vi "cross correlation trial.vi"() -> ()   [LabVIEW 2012, in "Thorcam.lvclass"]
uses:
  Thorcam.lvclass
  <vilib>/Analysis/baseanly.llb/Mean (DBL).vi
  <vilib>/vision/NI_Vision_Development_Module.lvlib
  <vilib>/Analysis/NI_AALBase.lvlib
panel:
  out "System XY Graph":cluster{i32[], i32[]}(graph)
  out "mean calculation time (ms)":dbl format="%0.2f"
  out "(x,y) of max":i32[](array[numeric])
  out "y axis average":sgl[](graph)
  out "x axis average":sgl[](graph)
  out "Rob":T1(plugin-control)
  out "Roy":T1(plugin-control)
  out "pixel position of max of CC":i32[](graph)
  out "error out":errorcluster
  out "CC":T1(plugin-control)
  in  "path 2":path
  in  "path":path
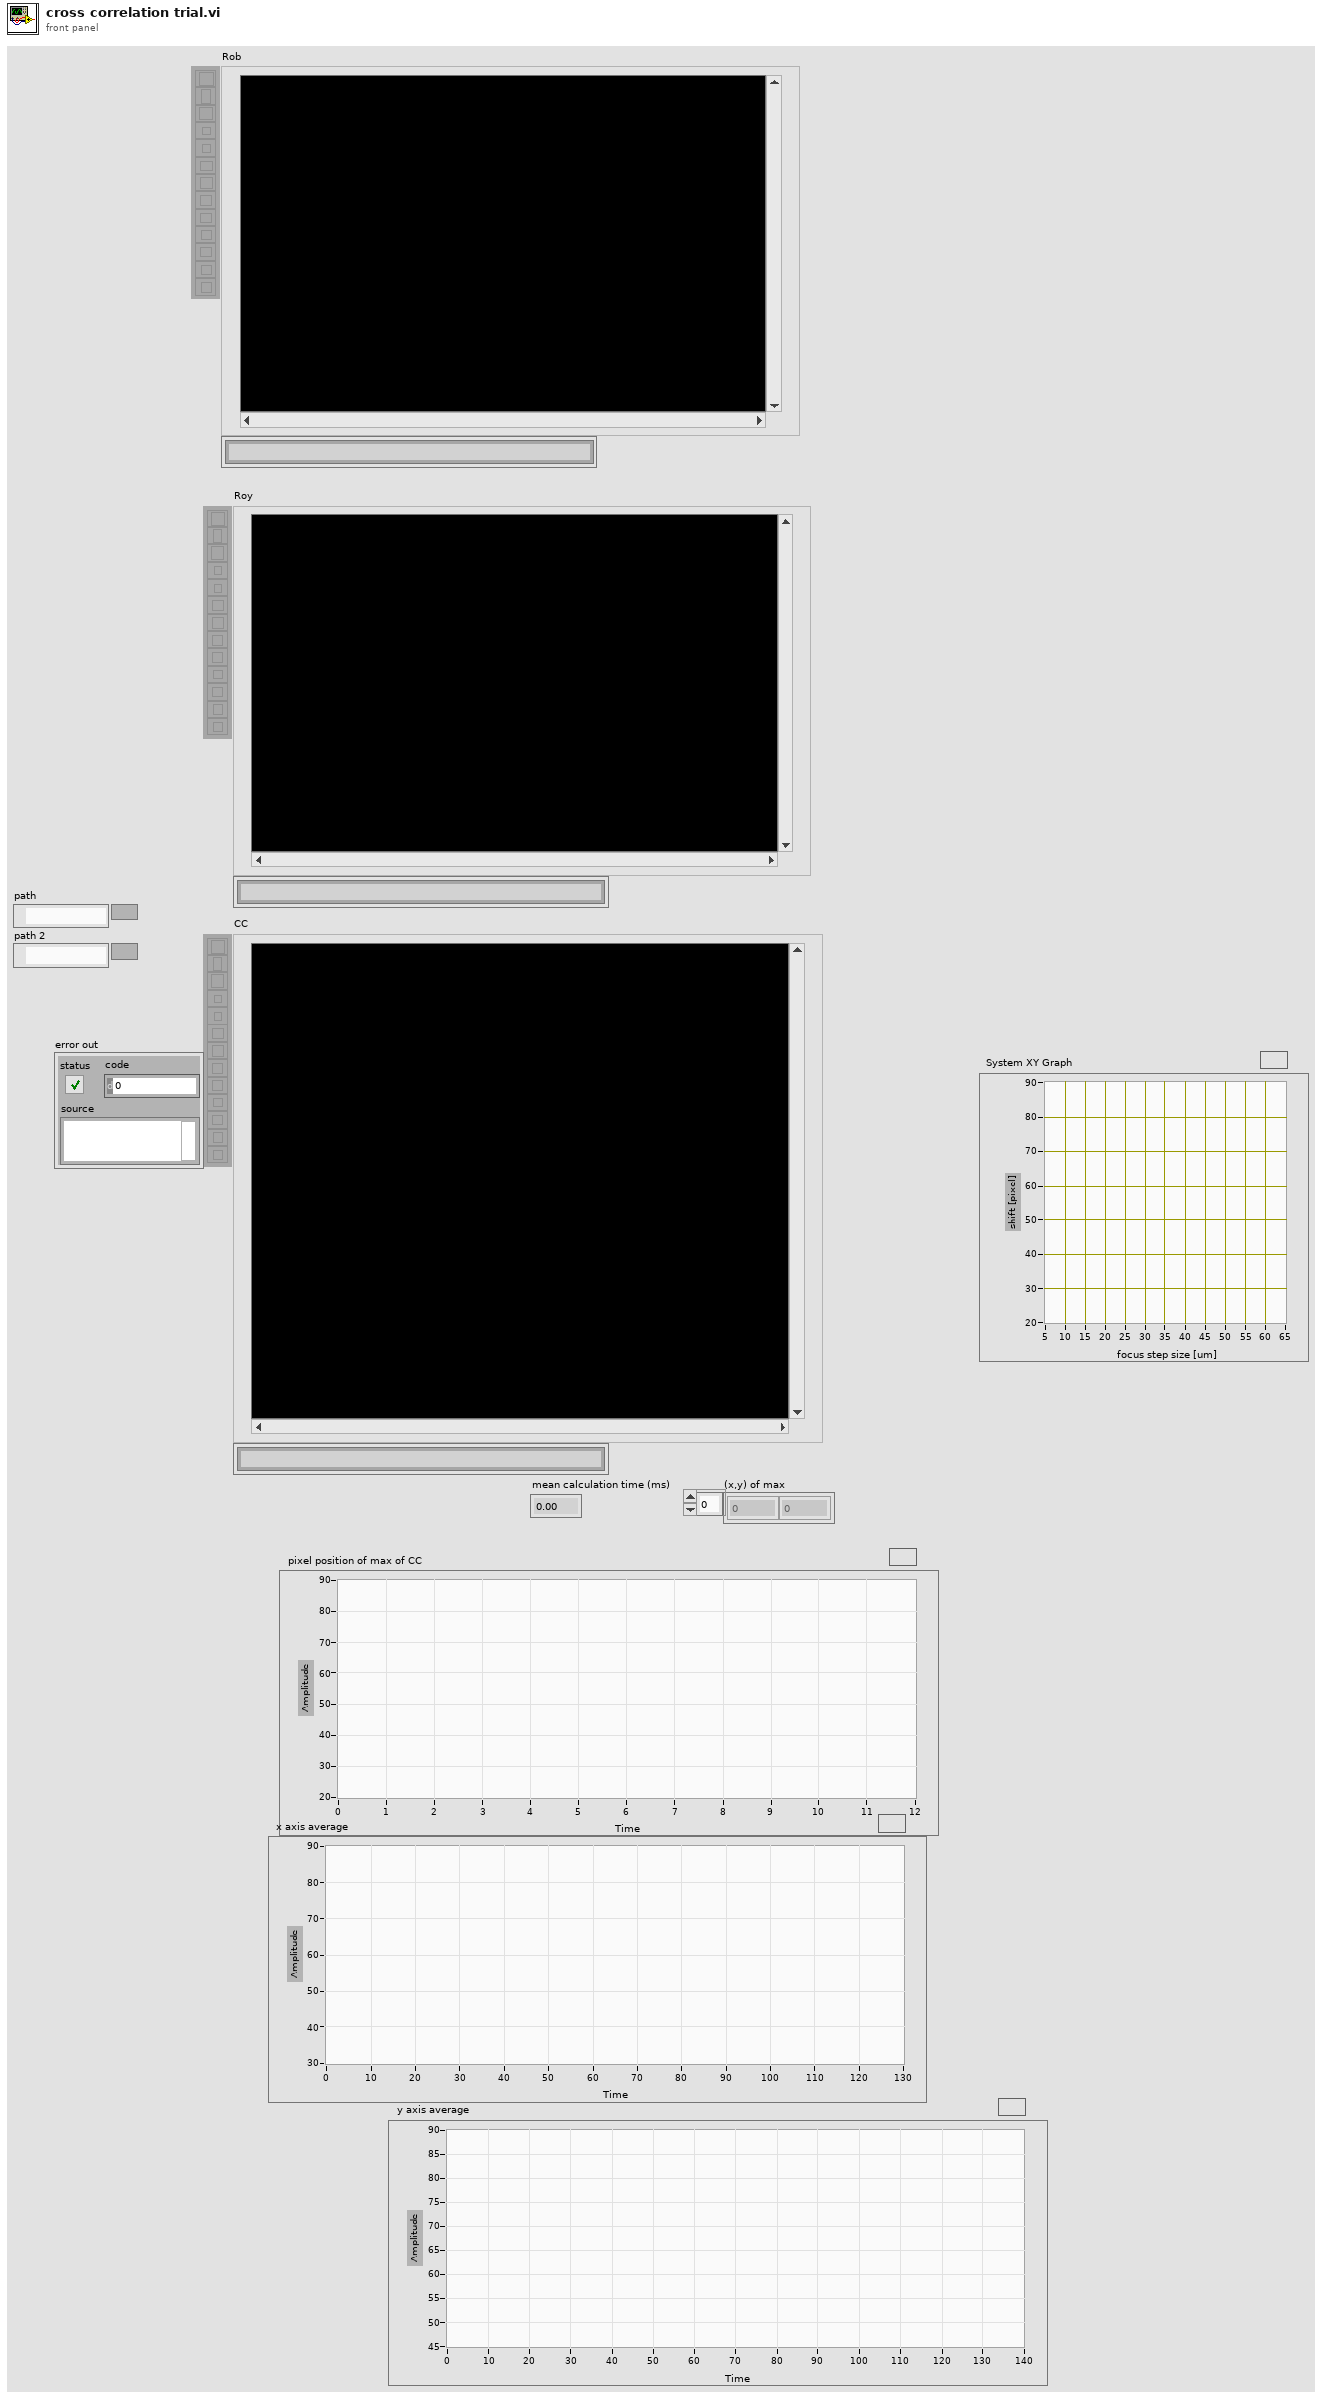
[diagram p1: front panel]
types:
  T1 = typedef "IMAQ Image.ctl" = refnum<image>
  T2 = cluster{"X Size":i32, "Y Size":i32, "Order #":i32}
  T3 = cluster{"histogram":u32[], "Minimal Value":sgl, "Maximal Value":sgl, "Starting Value":sgl, "Interval Width":sgl, "Mean Value":sgl, "Standard  Variation":sgl, "Area (pixels)":i32}
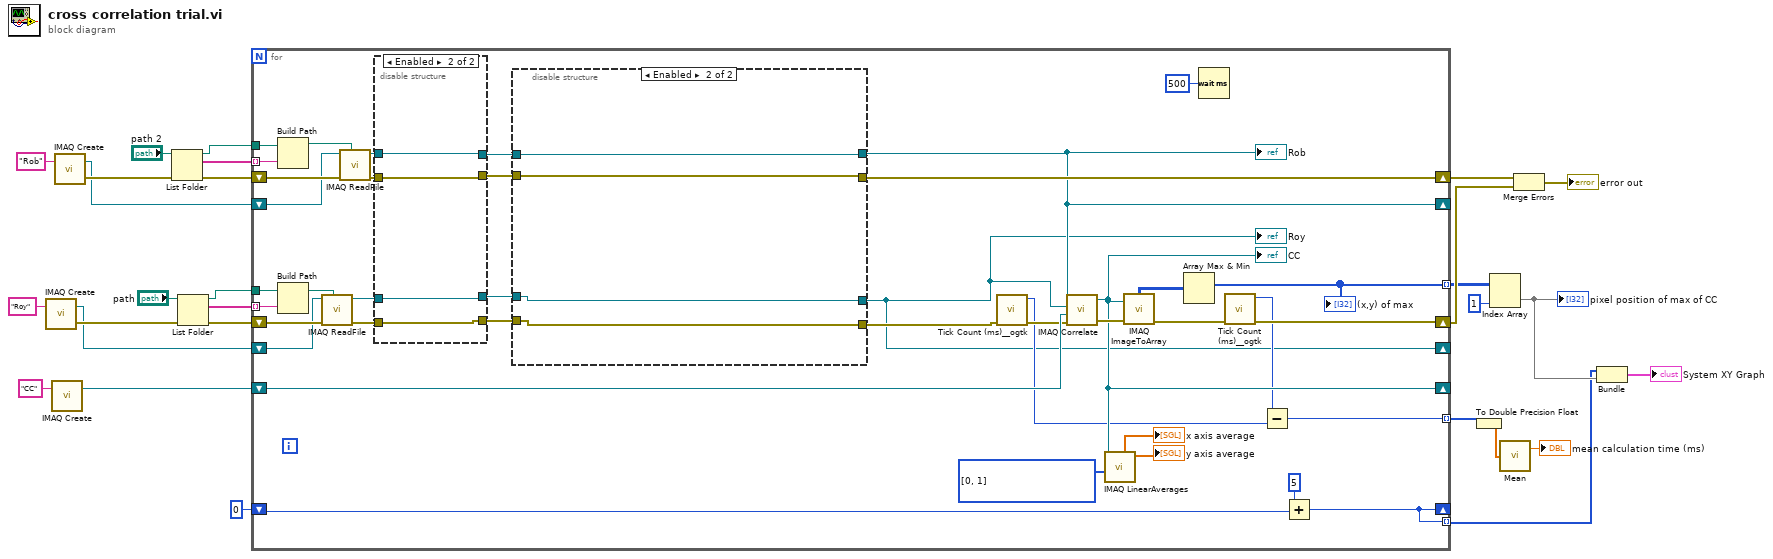
[diagram p0: block diagram]
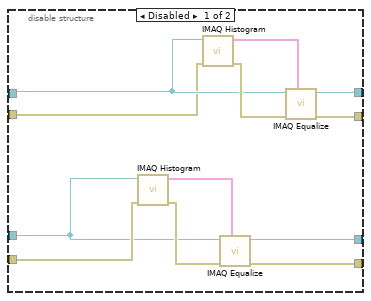
[diagram p2: hidden frame]
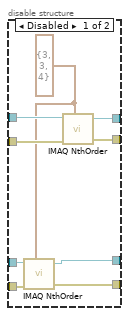
[diagram p3: hidden frame]
diagram:
  n1 = call "IMAQ Create"("Image Name"="Roy") -> ("New Image"=w18:T1, "error out"=w20:errorcluster)  [unwired: 4 in]
  n2 = call "IMAQ Create"("Image Name"="CC") -> ("New Image"=w10:T1)  [unwired: 4 in, 1 out]
  n3 = call "IMAQ Create"("Image Name"="Rob") -> ("New Image"=w21:T1, "error out"=w24:errorcluster)  [unwired: 4 in]
  n4 = List Folder(path="path 2", error in=w24) -> (path out=w22:path, filenames=w25:string[], error out=w23:errorcluster)  [unwired: 2 in, 1 out]
  n5 = List Folder(path="path", error in=w20) -> (path out=w17:path, filenames=w26:string[], error out=w19:errorcluster)  [unwired: 2 in, 1 out]
  n6 = for {
    tunnel: w26 -> [w61] mode=indexing
    tunnel: w25 -> [w67] mode=indexing
    tunnel: w22 -> [w66]
    shift-right: [w36] -> w14
    shift-left: w23 -> [w68]
    shift-right: [w35] -> _
    shift-left: w21 -> [w64]
    tunnel: w17 -> [w60]
    shift-right: [w47] -> w13
    shift-left: w19 -> [w63]
    shift-right: [w32] -> _
    shift-left: w18 -> [w62]
    tunnel: [w54] -> w9 mode=indexing
    shift-right: [w52] -> _
    shift-left: w10 -> [w55]
    tunnel: [w44] -> w7 mode=indexing
    shift-right: [w41] -> _
    shift-left: 0 -> [w42]
    tunnel: [w41] -> w2 mode=indexing
    w53 = i32[] [0, 1] items=["X Axis Averages", "Y Axis Averages", "X + Y Axis Averages", "X - Y Axis Averages"] ("Averages")
    n7 = Build Path(base path=w66, name or relative path=w67) -> (appended path=w65:path)
    n8 = Build Path(base path=w60, name or relative path=w61) -> (appended path=w59:path)
    n9 = call "IMAQ ReadFile"("File Path"=w59, "error in (no error)"=w63, "Image"=w62) -> ("error out"=w38:errorcluster, "Image Out"=w37:T1)  [unwired: 4 in, 3 out]
    n10 = call "IMAQ ReadFile"("File Path"=w65, "error in (no error)"=w68, "Image"=w64) -> ("error out"=w40:errorcluster, "Image Out"=w39:T1)  [unwired: 4 in, 3 out]
    n11 = disable-structure shown="Enabled" {
      disable-tunnel: w40 -> [w93 w96]
      disable-tunnel: w39 -> [w92 w97]
      disable-tunnel: w38 -> [w91 w94]
      disable-tunnel: w37 -> [w90 w95]
      disable-tunnel: [w88 w94] -> w34
      disable-tunnel: [w87 w95] -> w31
      disable-tunnel: [w86 w97] -> w30
      disable-tunnel: [w85 w96] -> w29
      frame Disabled {
        w89 = T2 {"X Size"=3, "Y Size"=3, "Order #"=4} ("Size & Order #")
        n12 = call "IMAQ NthOrder"("Image Src"=w90, "Size & Order #"=w89, "error in (no error)"=w91) -> ("Image Dst Out"=w87:T1, "error out"=w88:errorcluster)  [unwired: 4 in]
        n13 = call "IMAQ NthOrder"("Image Src"=w92, "Size & Order #"=w89, "error in (no error)"=w93) -> ("Image Dst Out"=w86:T1, "error out"=w85:errorcluster)  [unwired: 4 in]
      }
      frame Enabled {
      }
    }
    n14 = disable-structure shown="Enabled" {
      disable-tunnel: [w80 w83] -> w36
      disable-tunnel: [w79 w84] -> w35
      disable-tunnel: w34 -> [w76 w81]
      disable-tunnel: [w74 w81] -> w33
      disable-tunnel: [w72 w82] -> w32
      disable-tunnel: w31 -> [w71 w82]
      disable-tunnel: w30 -> [w70 w84]
      disable-tunnel: w29 -> [w69 w83]
      frame Disabled {
        n15 = call "IMAQ Histogram"("error in (no error)"=w76, "Image"=w71) -> ("error out"=w75:errorcluster, "Histogram Report"=w73:T3)  [unwired: 8 in]
        n16 = call "IMAQ Histogram"("error in (no error)"=w69, "Image"=w70) -> ("error out"=w78:errorcluster, "Histogram Report"=w77:T3)  [unwired: 8 in]
        n17 = call "IMAQ Equalize"("Histogram Report"=w73, "error in (no error)"=w75, "Image Src"=w71) -> ("error out"=w74:errorcluster, "Image Dst Out"=w72:T1)  [unwired: 7 in]
        n18 = call "IMAQ Equalize"("Histogram Report"=w77, "error in (no error)"=w78, "Image Src"=w70) -> ("error out"=w80:errorcluster, "Image Dst Out"=w79:T1)  [unwired: 7 in]
      }
      frame Enabled {
      }
    }
    "Roy" <- w32
    "Rob" <- w35
    n19 = call <userlib>:"Tick Count (ms)__ogtk.vi"("error in (no error)"=w33) -> ("error out"=w49:errorcluster, "millisecond timer value"=w45:u32)  [unwired: 9 in]
    n20 = call "IMAQ Correlate"("Image Src"=w35, "Image Template"=w32, "Image Dst"=w55, "error in (no error)"=w49) -> ("Image Dst Out"=w52:T1, "error out"=w58:errorcluster)  [unwired: 3 in]
    "CC" <- w52
    n21 = call "IMAQ LinearAverages"("Averages"=w53, "Image Src"=w52) -> ("Y Axis Averages"=→"y axis average":sgl[], "X Axis Averages"=→"x axis average":sgl[])  [unwired: 5 in, 3 out]
    n22 = call "IMAQ ImageToArray"("error in (no error)"=w58, "Image"=w52) -> ("error out"=w48:errorcluster, "Image Pixels (U8)"=w57:u8[][])  [unwired: 2 in, 3 out]
    n23 = Array Max & Min(array=w57) -> (max index (indices)=w54:i32[])  [unwired: 3 out]
    "(x,y) of max" <- w54
    n24 = Wait (ms)(milliseconds to wait=u32 500) -> ()  [unwired: 1 out]
    n25 = call <userlib>:"Tick Count (ms)__ogtk.vi"("error in (no error)"=w48) -> ("error out"=w47:errorcluster, "millisecond timer value"=w46:u32)  [unwired: 9 in]
    n26 = Subtract(x=w46, y=w45) -> (x-y=w44:u32)
    n27 = Add(x=5, y=w42) -> (x+y=w41:i32)
  }
  n28 = To Double Precision Float(number=w7) -> (double precision float=w5:dbl[])
  n29 = Index Array(array=w9, index (col)=1 ("disabled index (col)")) -> (element=w4:i32[])  [unwired: 1 in]
  "pixel position of max of CC" <- w4
  n30 = call-poly <vilib>:"Mean.vi"("X"=w5) -> ("mean"=→"mean calculation time (ms)":dbl)  [unwired: 1 out]
  n31 = Merge Errors(w14, w13) -> (→"error out":errorcluster)
  n32 = Bundle(w2, w4) -> (→"System XY Graph":cluster{i32[], i32[]})  [unwired: 1 in]
